vi "GetTerminals.vi"(6 "error in":errorcluster, 9 "Wire in":refnum<class "Wire.lvclass">) -> (0 "error out":errorcluster, 3 "Wire out":refnum<class "Wire.lvclass">, 4 "terminals":i32[](array[numeric]))   [LabVIEW 2014, in "Raspberry Pi Compatible Compiler for LabVIEW.lvlib" / "Wire.lvclass"]
uses:
  Wire.lvclass
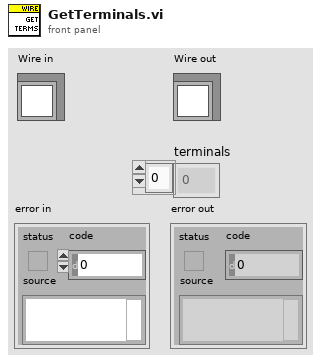
[diagram p1: front panel]
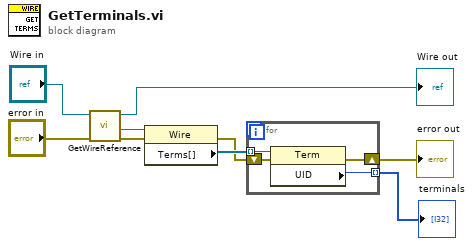
[diagram p0: block diagram]
diagram:
  n1 = call "GetWireReference.vi"("error in"="error in", "wire in"="Wire in") -> ("error out"=w7:errorcluster, "reference out"=w6:refnum<vi>, "wire out"=→"Wire out":refnum<class "Wire.lvclass">)  [unwired: 5 in]
  n2 = property class="Wire"(reference=w6, error in=w7) -> (error out=w3:errorcluster, "Terms[]"=w5:refnum<vi>[])  [unwired: 1 out]
  n3 = for {
    tunnel: w5 -> [w13] mode=indexing
    tunnel: [w12] -> w1 mode=indexing
    shift-right: [w10] -> w2
    shift-left: w3 -> [w11]
    n4 = property class="Term"(reference=w13, error in=w11) -> (error out=w10:errorcluster, "UID"=w12:i32)  [unwired: 1 out]
  }
  "error out" <- w2
  "terminals" <- w1
